vi "Logger.vi"() -> ()   [LabVIEW 2016]
uses:
  Logger.Action.ctl
  tools/CitTemplate/citTemplate.errData.ctl
  tools/EventLog/EventLog.EventSource.ctl
  Logger.FileBody.ctl
  Global/ApplicationGlobal.vi
panel:
  out "Folder":string
  out "_loop":i32(ring)=4
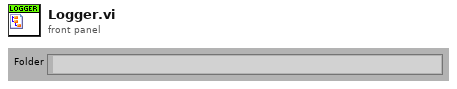
[diagram p1: front panel]
types:
  T1 = enum16{"open", "open or create", "create or replace", "create", "open (read-only)"}
  T2 = typedef "citTemplate.errData.ctl" = cluster{"ts":timestamp, "src":T3, "instance":i32, "action":string, "error":errorcluster, "unconfirmed":bool}
  T3 = typedef "EventLog.EventSource.ctl" = enum16{"All", "Gui", "Ref", "File", "Arch", "Seq", "CPX", "DB", "Laser", "Scan.P", "Scan.O"}
  T4 = typedef "Logger.FileBody.ctl" = cluster{"Path":path, "Status":u8, "Ref1":string, "Serial1":string, "Ref2":string, "Serial2":string, "Values":sgl[]}
  T5 = typedef "Logger.Action.ctl" = enum32{"idle", "constructor", "destructor", "--- Logger ---", "Begin", "Add", "End"}
  T6 = typedef "citTemplate.notifierHandle.ctl" = refnum<notifier>
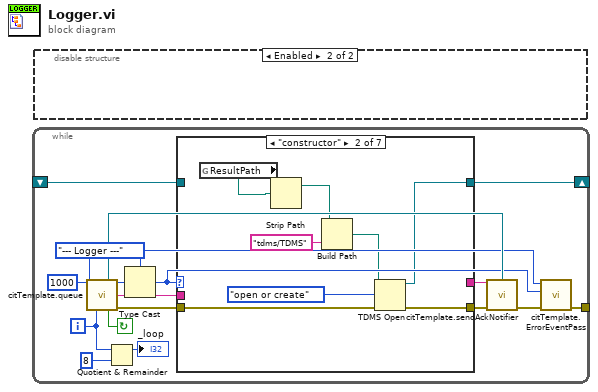
[diagram p0: block diagram]
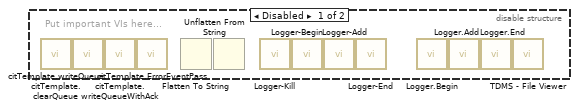
[diagram p2: hidden frame]
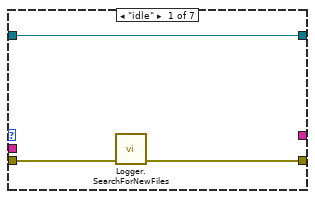
[diagram p3: hidden frame]
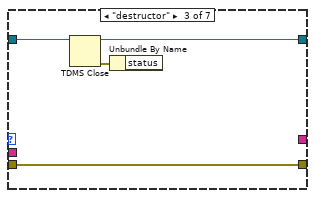
[diagram p4: hidden frame]
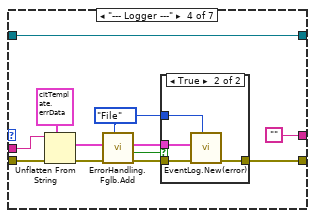
[diagram p5: hidden frame]
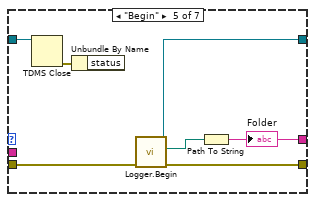
[diagram p7: hidden frame]
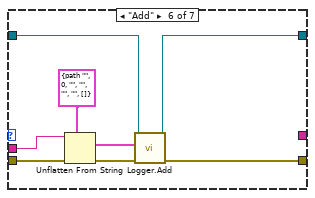
[diagram p8: hidden frame]
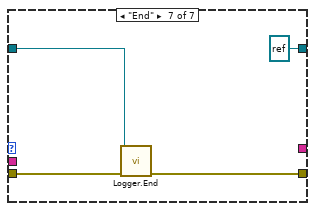
[diagram p9: hidden frame]
diagram:
  n1 = while {
    tunnel: [w4] -> _
    shift-right: [w2] -> _
    shift-left: _ -> [w1]
    i -> [w6]
    stop <- w13 continue-if-true
    w10 = Logger.Action."--- Logger ---" ("Action")
    n2 = call "citTemplate.queue.vi"("ms timeout (250 ms)"=1000, "event enum"=w10, "iteration (-1)"=w6) -> ("notifierHandle out"=w12:T6, "event out"=w16:u32, "(flatten) data out"=w15:string, "continue"=w13:bool, "error out"=w14:errorcluster)  [unwired: 2 in, 6 out]
    n3 = Quotient & Remainder(x=w6, y=8) -> (x-y*floor(x/y)=→"_loop":i32)  [unwired: 1 out]
    n4 = Type Cast(type=w10, x=w16) -> (*(type *) &x=w5:T5)
    n5 = case shown="\"constructor\"" w5 {
      tunnel: w15 -> [_ _ _ w40 _ w60 _]
      tunnel: w14 -> [w18 w26 w30 w39 w47 w61 w62]
      tunnel: [_ _ _ "" w48 _ _] -> w11
      tunnel: [w17 w25 w30 w32 w53 w58 w63] -> w9
      tunnel: [w19 w27 w29 w31 w50 w56 refnum<k34> refnum ("Refnum out")] -> w2
      tunnel: w1 -> [w19 _ w29 w31 w52 w57 w65]
      frame "idle" {
        n6 = call "Logger.SearchForNewFiles.vi"("error in"=w18) -> ("error out"=w17:errorcluster)  [unwired: 10 in]
      }
      frame "constructor" {
        n7 = global read "ApplicationGlobal.vi" "ResultPath"() -> (w23:path)
        n8 = Strip Path(path=w23) -> (stripped path=w22:path)  [unwired: 1 out]
        n9 = Build Path(base path=w22, name or relative path="tdms/TDMS") -> (appended path=w21:path)
        n10 = TDMS Open(8:w26, 10:T1."open or create" ("operation (0:open)"), 11:w21) -> (0:w25:errorcluster, 3:w27:refnum<k34>)  [unwired: 4 in]
      }
      frame "destructor" {
        n11 = TDMS Close(11:w29) -> (0:w28:errorcluster)  [unwired: 1 in, 1 out]
        n12 = Unbundle By Name(w28) -> ()  [unwired: 1 out]
      }
      frame "--- Logger ---" {
        w33 = EventLog.EventSource."File" ("Event source")
        n13 = Unflatten From String(type=T2 {"ts"=timestamp(0 s since 1904-01-01), "src"=enum."All", "instance"=0, "action"="", "error"={"status"=FALSE, "code"=0, "source"=""}, "unconfirmed"=FALSE} ("ErrData"), binary string=w40, error in (no error)=w39) -> (value=w34:T2, error out=w35:errorcluster)  [unwired: 3 out]
        n14 = call "ErrorHandling.Fglb.Add.vi"("Event source"=w33, "error in (no error)"=w35, "Error in"=w34) -> ("error out"=w37:errorcluster, "changed?"=w36:bool)  [unwired: 7 in]
        n15 = case shown="True" w36 {
          tunnel: [w42 w46] -> w32
          tunnel: w34 -> [_ w45]
          tunnel: w37 -> [w42 w44]
          tunnel: w33 -> [_ w43]
          frame False {
          }
          frame True {
            n16 = call "EventLog.New(error).vi"("Source (All)"=w43, "error in"=w44, "ErrData"=w45) -> ("error out"=w46:errorcluster)  [unwired: 8 in]
          }
        }
      }
      frame "Begin" {
        n17 = TDMS Close(11:w52) -> (0:w51:errorcluster)  [unwired: 1 in, 1 out]
        n18 = Unbundle By Name(w51) -> ()  [unwired: 1 out]
        n19 = call "Logger.Begin.vi"("error in"=w47) -> ("error out"=w53:errorcluster, "Folder"=w49:path, "Refnum out"=w50:refnum<k34>)  [unwired: 8 in]
        n20 = Path To String(path=w49) -> (string=w48:string)
        "Folder" <- w48
      }
      frame "Add" {
        n21 = Unflatten From String(type=T4 {"Path"=path "", "Status"=0, "Ref1"="", "Serial1"="", "Ref2"="", "Serial2"="", "Values"=[]} ("PLCvalues"), binary string=w60, error in (no error)=w61) -> (value=w55:T4, error out=w59:errorcluster)  [unwired: 3 out]
        n22 = call "Logger.Add.vi"("error in"=w59, "HandledFileContent"=w55, "Refnum in"=w57) -> ("error out"=w58:errorcluster, "Refnum out"=w56:refnum<k34>)  [unwired: 7 in]
      }
      frame "End" {
        n23 = call "Logger.End.vi"("error in"=w62, "Refnum in"=w65) -> ("error out"=w63:errorcluster)  [unwired: 8 in, 1 out]
      }
    }
    n24 = call "citTemplate.sendAckNotifier.vi"("notification data"=w11, "notifierHandle in"=w12, "error in"=w9) -> ()  [unwired: 13 out]
    n25 = call "citTemplate.ErrorEventPass.vi"("error in"=w9, "action of error"=w5, "event in"=w10) -> ("error out"=w4:errorcluster)  [unwired: 2 in, 6 out]
  }
  n26 = disable-structure shown="Enabled" {
    frame Disabled {
      # "Put important VIs here..."
      n27 = call "citTemplate.clearQueue.vi"() -> ()  [unwired: 14 in, 2 out]
      n28 = call "citTemplate.writeQueue.vi"() -> ()  [unwired: 15 in, 1 out]
      n29 = call "citTemplate.writeQueueWithAck.vi"() -> ()  [unwired: 13 in, 3 out]
      n30 = call "citTemplate.ErrorEventPass.vi"() -> ()  [unwired: 11 in, 1 out]
      n31 = Flatten To String() -> ()  [unwired: 4 in, 3 out]
      n32 = Unflatten From String() -> ()  [unwired: 5 in, 3 out]
      n33 = call "Logger-Kill.vi"() -> ()  [unwired: 11 in, 1 out]
      n34 = call "Logger-Begin.vi"() -> ()  [unwired: 10 in, 2 out]
      n35 = call "Logger-Add.vi"() -> ()  [unwired: 11 in, 1 out]
      n36 = call "Logger-End.vi"() -> ()  [unwired: 11 in, 1 out]
      n37 = call "Logger.Begin.vi"() -> ()  [unwired: 9 in, 3 out]
      n38 = call "Logger.Add.vi"() -> ()  [unwired: 10 in, 2 out]
      n39 = call "Logger.End.vi"() -> ()  [unwired: 10 in, 2 out]
      n40 = call <vilib>:"TDMS - File Viewer.vi"() -> ()  [unwired: 6 in, 2 out]
    }
    frame Enabled {
    }
  }
